vi "Write Keepalive.vi"(8 "error in (no error)":errorcluster, 10 "Keepalive":T1={"Enabled"=FALSE, "Ping Interval (ms)"=25000, "Ping Timeout (ms)"=20000}, 11 "WS Test Client Subscriber in":refnum<class "WS Test Client Subscriber.lvclass">) -> (0 "error out":errorcluster, 3 "WS Test Client Subscriber out":refnum<class "WS Test Client Subscriber.lvclass">)   [LabVIEW 2021, in "Echo Reply Test With Server Manager.lvlib" / "WS Test Client Subscriber.lvclass"]
uses:
  WS Test Client Subscriber.lvclass
  WS Test Client Subscriber.lvclass/WS Test Client Subscriber.ctl
  WebSocket Actor/WebSocket Connection/Keepalive.ctl
  WebSocket Actor/WebSocket Connection/WebSocket Connection.lvclass
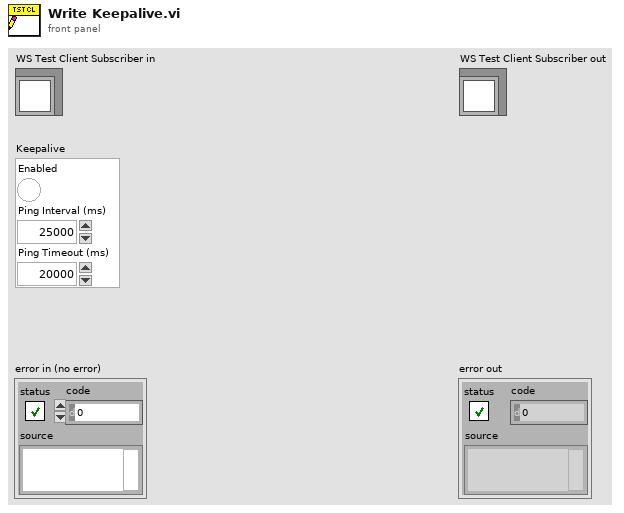
[diagram p1: front panel]
types:
  T1 = typedef "WebSocket Actors.lvlib/WebSocket Connection.lvclass/Keepalive.ctl" = cluster{"Enabled":bool, "Ping Interval (ms)":u32, "Ping Timeout (ms)":u32}
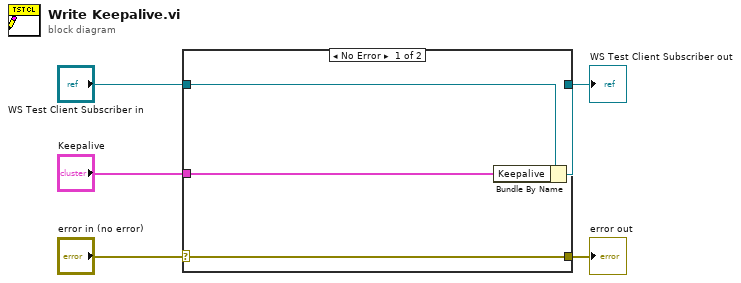
[diagram p0: block diagram]
diagram:
  n1 = case shown="No Error" "error in (no error)" {
    selector: "error in (no error)" -> [w9 w10]
    tunnel: [w9 w10] -> w4
    tunnel: [w7 w11] -> w2
    tunnel: "WS Test Client Subscriber in" -> [w8 w11]
    tunnel: "Keepalive" -> [w6 _]
    frame No Error {
      n2 = Bundle By Name(cluster=w8, "Keepalive"=w6) -> (w7:refnum<class "WS Test Client Subscriber.lvclass">)
    }
    frame Error {
    }
  }
  "error out" <- w4
  "WS Test Client Subscriber out" <- w2
